vi "Write Sub-Menus.vi"(8 "error in (no error)":errorcluster, 10 "Menu Items":refnum<data-value>[](array[refnum]), 11 "MGI_MenuItem in":refnum<class "MGI_MenuItem.lvclass">) -> (0 "error out":errorcluster, 3 "MGI_MenuItem out":refnum<class "MGI_MenuItem.lvclass">)   [LabVIEW 2016, in "MGI_MenuItem.lvclass"]
doc: "Sub-menus are expanded out from the menu item when the item is highlighted. A menu item with submenus cannot be clicked by the user, although it can be clicked programatically.\n\nAuthored by Derek E. Trepanier\nsupport@mooregoodideas.com\nwww.mooregoodideas.com\n\nCopyright (c) 2012, Moore Good Ideas, Inc.\n\nAll rights reserved.\n\nRedistribution and use in source and binary forms, with or without modification, are permitted provided that the following conditions are met:\n\n * Redistributions of source code must retain the above copyright notice, this list of conditions and the following disclaimer.\n * Redistributions in binary form must reproduce the above copyright notice, this list of conditions and the following disclaimer in the documentation and/or other materials provided with the distribution.\n * Neither the name of Moore Good Ideas, Inc. nor the names of its contributors may be used to endorse or promote products derived from this software without specific prior written permission.\n\nTHIS SOFTWARE IS PROVIDED BY THE COPYRIGHT HOLDERS AND CONTRIBUTORS \"AS IS\" AND ANY EXPRESS OR IMPLIED WARRANTIES, INCLUDING, BUT NOT LIMITED TO, THE IMPLIED WARRANTIES OF MERCHANTABILITY AND FITNESS FOR A PARTICULAR PURPOSE ARE DISCLAIMED. IN NO EVENT SHALL THE COPYRIGHT OWNER OR CONTRIBUTORS BE LIABLE FOR ANY DIRECT, INDIRECT, INCIDENTAL, SPECIAL, EXEMPLARY, OR CONSEQUENTIAL DAMAGES (INCLUDING, BUT NOT LIMITED TO, PROCUREMENT OF SUBSTITUTE GOODS OR SERVICES; LOSS OF USE, DATA, OR PROFITS; OR BUSINESS INTERRUPTION) HOWEVER CAUSED AND ON ANY THEORY OF LIABILITY, WHETHER IN CONTRACT, STRICT LIABILITY, OR TORT (INCLUDING NEGLIGENCE OR OTHERWISE) ARISING IN ANY WAY OUT OF THE USE OF THIS SOFTWARE, EVEN IF ADVISED OF THE POSSIBILITY OF SUCH DAMAGE."
uses:
  <userlib>/_MGI/Menu Building/MenuItem/MGI_MenuItem.lvclass
  <userlib>/_MGI/Menu Building/MenuItem/MGI_MenuItem.lvclass/MGI_MenuItem.ctl
  <userlib>/_MGI/Menu Building/MenuItem/Read Tag.vi
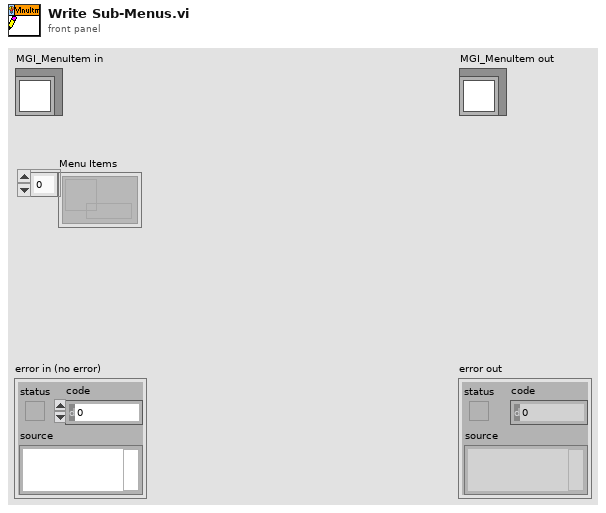
[diagram p1: front panel]
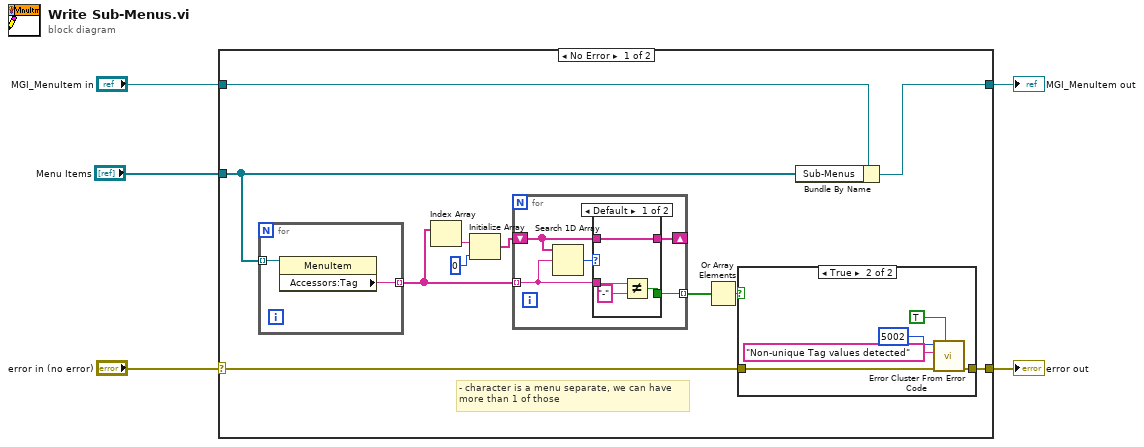
[diagram p0: block diagram]
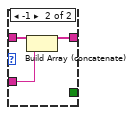
[diagram p3: hidden frame]
diagram:
  n1 = case shown="No Error" "error in (no error)" {
    selector: "error in (no error)" -> [w7 w37]
    tunnel: [w6 w37] -> w4
    tunnel: [w15 w38] -> w2
    tunnel: "MGI_MenuItem in" -> [w16 w38]
    tunnel: "Menu Items" -> [w10 _]
    frame No Error {
      # "- character is a menu separate, we can have\nmore than 1 of those"
      n2 = for {
        tunnel: w10 -> [w36] mode=indexing
        tunnel: [w35] -> w11 mode=indexing
        n3 = property class="MenuItem"(reference=w36) -> ("Accessors:Tag"=w35:string)  [unwired: 1 in, 2 out]
      }
      n4 = Index Array(array=w11) -> (element=w14:string)  [unwired: 1 in]
      n5 = Initialize Array(w14, 0 ("Dimension Size")) -> (w13:string[])
      n6 = for {
        tunnel: w11 -> [w26] mode=indexing
        shift-right: [w25] -> _
        shift-left: w13 -> [w24]
        tunnel: [w23] -> w9 mode=indexing
        n7 = Search 1D Array(1D array=w24, element=w26) -> (index of element=w27:i32)  [unwired: 1 in]
        n8 = case shown="Default" w27 {
          tunnel: w26 -> [w29 w34]
          tunnel: [w31 w32] -> w25
          tunnel: w24 -> [w31 w33]
          tunnel: [w30 _] -> w23
          frame Default {
            n9 = Not Equal?(x=w29, y="-") -> (x != y?=w30:bool)
          }
          frame -1 {
            n10 = Build Array (concatenate)(w33, w34) -> (w32:string[])
          }
        }
      }
      n11 = Or Array Elements(Boolean array=w9) -> (logical OR=w8:bool)
      n12 = case shown="True" w8 {
        tunnel: w7 -> [w17 w22]
        tunnel: [w17 w21] -> w6
        frame False {
        }
        frame True {
          n13 = call <vilib>:"Error Cluster From Error Code.vi"("show call chain? (False)"=TRUE, "error in (no error)"=w22, "error message (\"\")"="Non-unique Tag values detected" ("error message (\"\")"), "error code (0)"=5002) -> ("error out"=w21:errorcluster)  [unwired: 5 in]
        }
      }
      n14 = Bundle By Name(cluster=w16, "Sub-Menus"=w10) -> (w15:refnum<class "MGI_MenuItem.lvclass">)
    }
    frame Error {
    }
  }
  "error out" <- w4
  "MGI_MenuItem out" <- w2
